vi "Scanning Variables.vi"() -> ()   [LabVIEW 2018]
panel:
  out "?":string
  out "?":string
  out "?":string
  out "?":string
  out "?":string
  out "?":string
  out "?":string
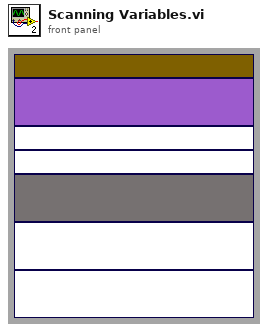
[diagram p1: front panel]
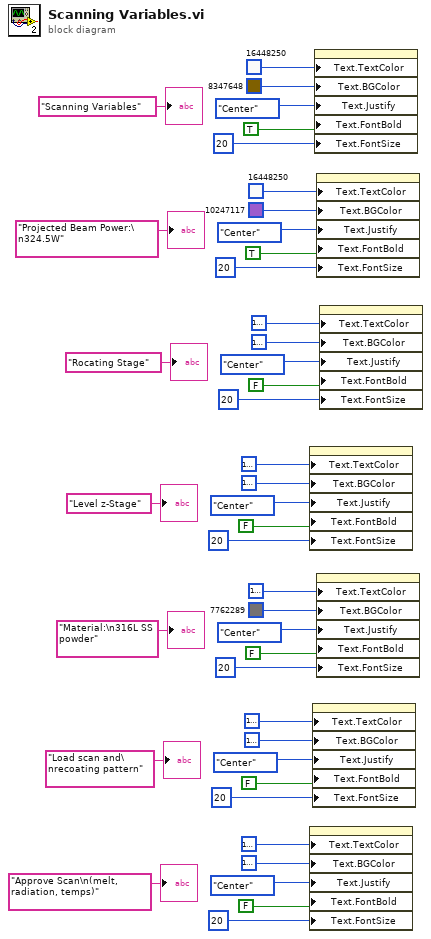
[diagram p0: block diagram]
diagram:
  n1 = property class="Str"("Text.TextColor"=u32 16777222, "Text.BGColor"=u32 16777226, "Text.Justify"=enum16{"Left", "Center", "Right"}."Center" ("Text.Justification"), "Text.FontBold"=FALSE ("Text.Font:Bold"), "Text.FontSize"=u32 20 ("Text.Font:Size")) -> ()  [unwired: 2 in, 2 out]
  n2 = property class="Str"("Text.TextColor"=u32 16777222, "Text.BGColor"=u32 16777226, "Text.Justify"=enum16{"Left", "Center", "Right"}."Center" ("Text.Justification"), "Text.FontBold"=FALSE ("Text.Font:Bold"), "Text.FontSize"=u32 20 ("Text.Font:Size")) -> ()  [unwired: 2 in, 2 out]
  n3 = property class="Str"("Text.TextColor"=u32 16777222, "Text.BGColor"=u32 16777226, "Text.Justify"=enum16{"Left", "Center", "Right"}."Center" ("Text.Justification"), "Text.FontBold"=FALSE ("Text.Font:Bold"), "Text.FontSize"=u32 20 ("Text.Font:Size")) -> ()  [unwired: 2 in, 2 out]
  n4 = property class="Str"("Text.TextColor"=u32 16448250, "Text.BGColor"=u32 8347648, "Text.Justify"=enum16{"Left", "Center", "Right"}."Center" ("Text.Justification"), "Text.FontBold"=TRUE ("Text.Font:Bold"), "Text.FontSize"=u32 20 ("Text.Font:Size")) -> ()  [unwired: 2 in, 2 out]
  n5 = property class="Str"("Text.TextColor"=u32 16448250, "Text.BGColor"=u32 10247117, "Text.Justify"=enum16{"Left", "Center", "Right"}."Center" ("Text.Justification"), "Text.FontBold"=TRUE ("Text.Font:Bold"), "Text.FontSize"=u32 20 ("Text.Font:Size")) -> ()  [unwired: 2 in, 2 out]
  n6 = property class="Str"("Text.TextColor"=u32 16777238, "Text.BGColor"=u32 7762289, "Text.Justify"=enum16{"Left", "Center", "Right"}."Center" ("Text.Justification"), "Text.FontBold"=FALSE ("Text.Font:Bold"), "Text.FontSize"=u32 20 ("Text.Font:Size")) -> ()  [unwired: 2 in, 2 out]
  n7 = property class="Str"("Text.TextColor"=u32 16777222, "Text.BGColor"=u32 16777226, "Text.Justify"=enum16{"Left", "Center", "Right"}."Center" ("Text.Justification"), "Text.FontBold"=FALSE ("Text.Font:Bold"), "Text.FontSize"=u32 20 ("Text.Font:Size")) -> ()  [unwired: 2 in, 2 out]
  "?" <- "Projected Beam Power:\n324.5W" ("String")
  "?" <- "Scanning Variables" ("String")
  "?" <- "Rocating Stage" ("String")
  "?" <- "Level z-Stage" ("String")
  "?" <- "Material:\n316L SS powder" ("String")
  "?" <- "Load scan and\nrecoating pattern" ("String")
  "?" <- "Approve Scan\n(melt, radiation, temps)" ("String")
